vi "Recent VIs - DataStorage.vi"(0 "Current VIs - Data":T1, 5 "Search VI Name":string, 7 "No. Data To Store":i32, 11 "error in (no error)":errorcluster, 12 "Operation":T3(ring)) -> (4 "AllDataInStorage":T1[](array[typedef]), 6 "IndexOfFoundData":i32, 10 "Found?":bool, 15 "error out":errorcluster)   [LabVIEW 2014, in "SmartPalette.lvlib"]
uses:
  SmartPalette.lvlib
  Controls/VI - DataStorage.ctl
  Controls/GObjectDetail.ctl
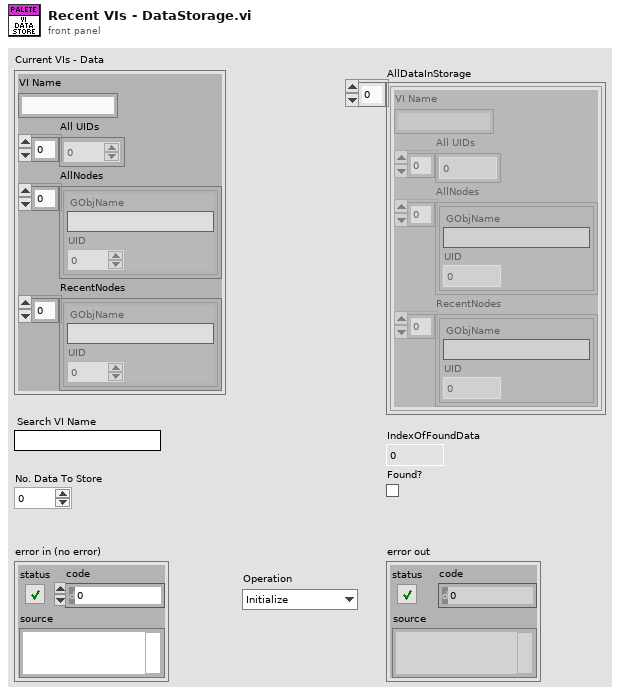
[diagram p1: front panel]
types:
  T1 = typedef "SmartPalette.lvlib/VI - DataStorage.ctl" = cluster{"VI Name":string, "All UIDs":i32[], "AllNodes":T2[], "RecentNodes":T2[]}
  T2 = typedef "SmartPalette.lvlib/GObjectDetail.ctl" = cluster{"GObjName":string, "UID":i32}
  T3 = enum16{"Initialize", "StoreData", "Serach&GetData", "DeleteAll"}
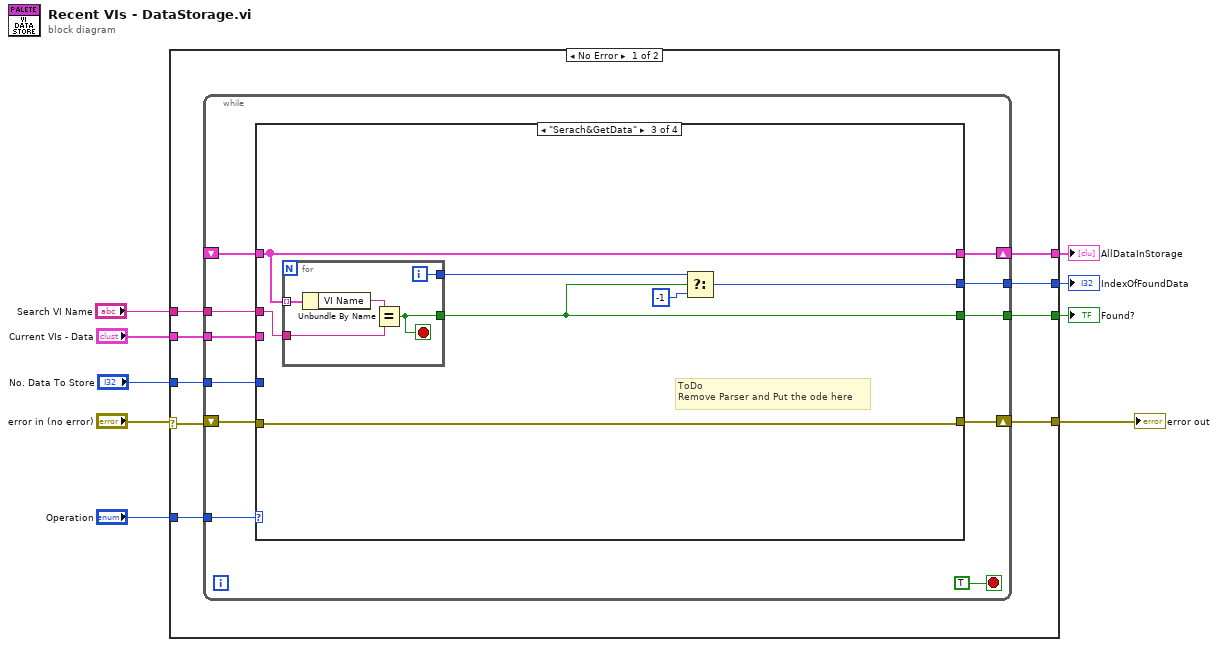
[diagram p0: block diagram]
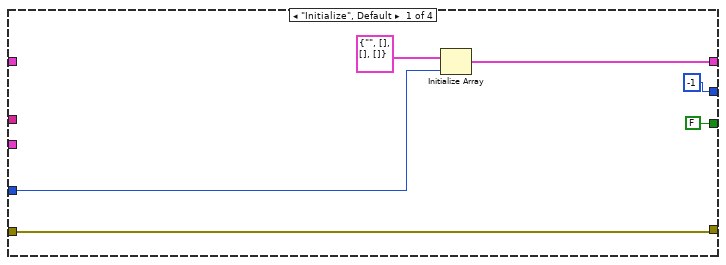
[diagram p2: hidden frame]
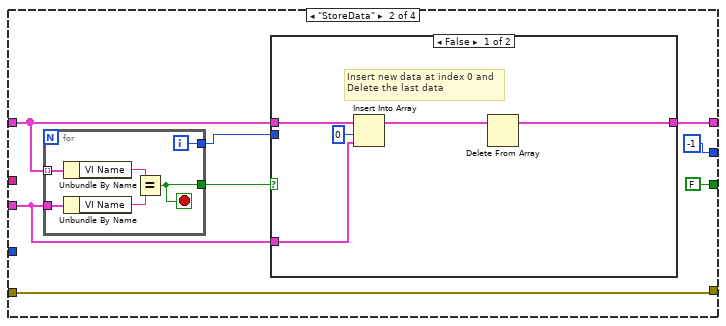
[diagram p3: hidden frame]
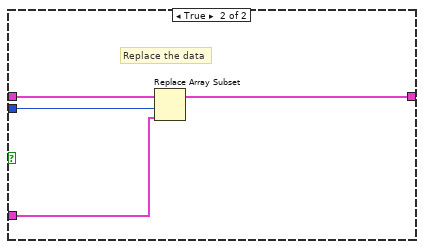
[diagram p4: hidden frame]
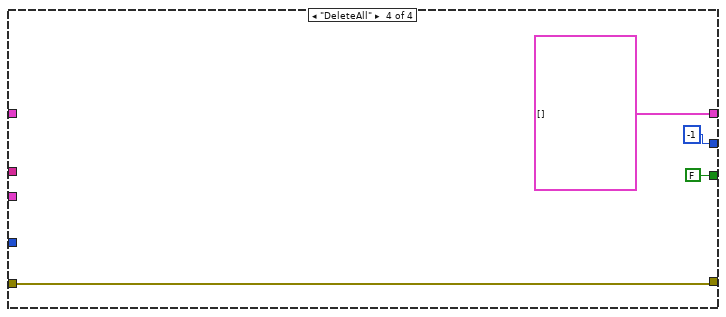
[diagram p5: hidden frame]
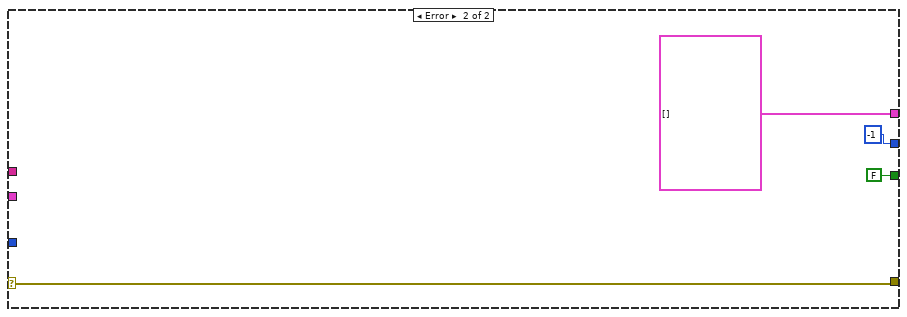
[diagram p6: hidden frame]
diagram:
  n1 = case shown="No Error" "error in (no error)" {
    selector: "error in (no error)" -> [w14 w78]
    tunnel: [w18 w78] -> w8
    tunnel: "Operation" -> [w17 _]
    tunnel: "No. Data To Store" -> [w16 _]
    tunnel: [w15 T1[] []] -> w5
    tunnel: "Current VIs - Data" -> [w13 _]
    tunnel: "Search VI Name" -> [w12 _]
    tunnel: [w11 -1] -> w2
    tunnel: [w10 FALSE] -> w1
    frame No Error {
      n2 = while {
        tunnel: w17 -> [w27]
        shift-right: [w28] -> w18
        shift-left: w14 -> [w29]
        tunnel: w16 -> [w25]
        shift-right: [w24] -> w15
        shift-left: _ -> [w23]
        tunnel: w13 -> [w22]
        tunnel: w12 -> [w21]
        tunnel: [w20] -> w11
        tunnel: [w19] -> w10
        stop <- TRUE stop-if-true
        n3 = case shown="\"Serach&GetData\"" w27 {
          tunnel: w29 -> [w32 w43 w64 w71]
          tunnel: [w32 w43 w64 w71] -> w28
          tunnel: w25 -> [w34 _ _ _]
          tunnel: [w33 w39 w63 T1[] []] -> w24
          tunnel: w23 -> [_ w40 w63 _]
          tunnel: w22 -> [_ w38 _ _]
          tunnel: w21 -> [_ _ w65 _]
          tunnel: [-1 -1 w60 -1] -> w20
          tunnel: [FALSE FALSE w61 FALSE] -> w19
          frame "Initialize", Default {
            n4 = Initialize Array(T1 {"VI Name"="", "All UIDs"=[], "AllNodes"=[], "RecentNodes"=[]} ("Current VIs - DataStorage"), w34) -> (w33:T1[])
          }
          frame "StoreData" {
            n5 = for {
              tunnel: w40 -> [w58] mode=indexing
              tunnel: w38 -> [w57]
              tunnel: [w54] -> w42
              tunnel: [w53] -> w41
              i -> [w53]
              stop <- w54 stop-if-true
              n6 = Unbundle By Name(w58) -> ("VI Name"=w56:string)
              n7 = Unbundle By Name(w57) -> ("VI Name"=w55:string)
              n8 = Equal?(x=w56, y=w55) -> (x = y?=w54:bool)
            }
            n9 = case shown="False" w42 {
              tunnel: w41 -> [_ w50]
              tunnel: w40 -> [w48 w52]
              tunnel: [w46 w51] -> w39
              tunnel: w38 -> [w45 w49]
              frame False {
                # "Insert new data at index 0 and\nDelete the last data"
                n10 = Insert Into Array(array=w48, index=0, new element=w45) -> (w47:T1[])
                n11 = Delete From Array(array=w47) -> (array with subset deleted=w46:T1[])  [unwired: 2 in, 1 out]
              }
              frame True {
                # "Replace the data"
                n12 = Replace Array Subset(array=w52, new element=w49, index=w50) -> (w51:T1[])
              }
            }
          }
          frame "Serach&GetData" {
            # "ToDo\nRemove Parser and Put the ode here"
            n13 = for {
              tunnel: w63 -> [w70] mode=indexing
              tunnel: [w68] -> w61
              tunnel: [w67] -> w62
              tunnel: w65 -> [w66]
              i -> [w67]
              stop <- w68 stop-if-true
              n14 = Unbundle By Name(w70) -> ("VI Name"=w69:string)
              n15 = Equal?(x=w69, y=w66) -> (x = y?=w68:bool)
            }
            n16 = Select(t=w62, s=w61, f=-1) -> (s? t:f=w60:i32)
          }
          frame "DeleteAll" {
          }
        }
      }
    }
    frame Error {
    }
  }
  "error out" <- w8
  "AllDataInStorage" <- w5
  "IndexOfFoundData" <- w2
  "Found?" <- w1
